vi "Creation IHM Affiche Result.vi"(8 "error in (no error)":errorcluster caption="entrée d'erreur (pas d'erreur)", 10 "Test Result":T3(array[cluster]), 11 "Arbre Liste SN":refnum<vi>) -> (0 "error out":errorcluster caption="sortie d'erreur")   [LabVIEW 2020, in "Library Instrument & Equipement.lvlib" / "Library Popup.lvlib" / "Class Popup Result_Info (Virtual).lvclass"]
uses:
  Class Popup Result_Info (Virtual).lvclass
  Commun VI/TypeDef/Commande Test/Commande Value Type.ctl
  Commun VI/TypeDef/Commande Test/Commande Type Test.ctl
  Commun VI/Library Commun.lvlib
panel:
  in  "Tableau élément":T4(array[cluster])
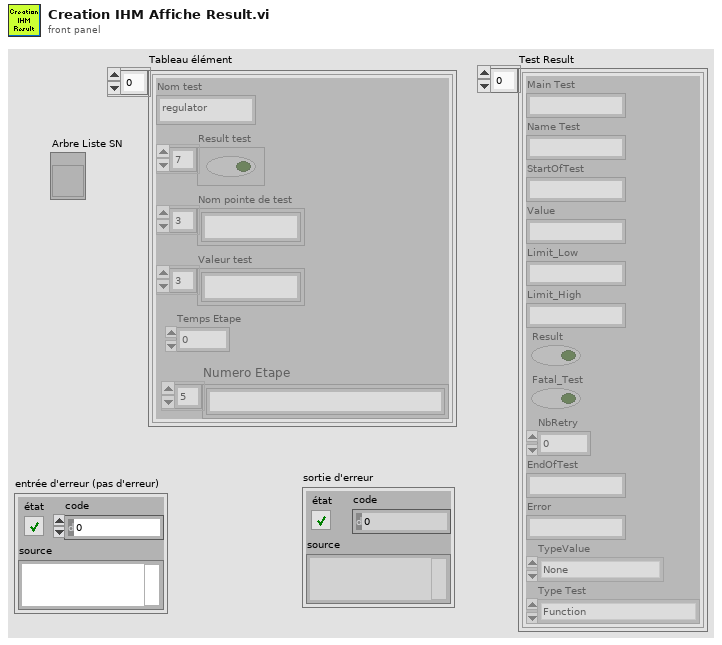
[diagram p1: front panel]
types:
  T1 = typedef "Library Commun.lvlib/Commande Value Type.ctl" = enum16{"None", "String", "Number", "Timestamp", "Boolean", "Array"}
  T2 = typedef "Library Commun.lvlib/Commande Type Test.ctl" = enum16{"Function", "Test", "Calculation"}
  T3 = cluster{"Main Test":string, "Name Test":string, "StartOfTest":string, "Value":string, "Limit_Low":string, "Limit_High":string, "Result":bool, "Fatal_Test":bool, "NbRetry":dbl, "EndOfTest":string, "Error":string, "TypeValue":T1, "Type Test":T2}[]
  T4 = cluster{"Nom test":string, "Result test":bool[], "Nom pointe de test":string[], "Valeur test":string[], "Temps Etape":dbl, "Numero Etape":string[]}[]
  T5 = cluster{"Main Test":string, "Name Test":string, "StartOfTest":string, "Value":string, "Limit_Low":string, "Limit_High":string, "Result":bool, "Fatal_Test":bool, "NbRetry":dbl, "EndOfTest":string, "Error":string, "TypeValue":T1, "Type Test":T2}
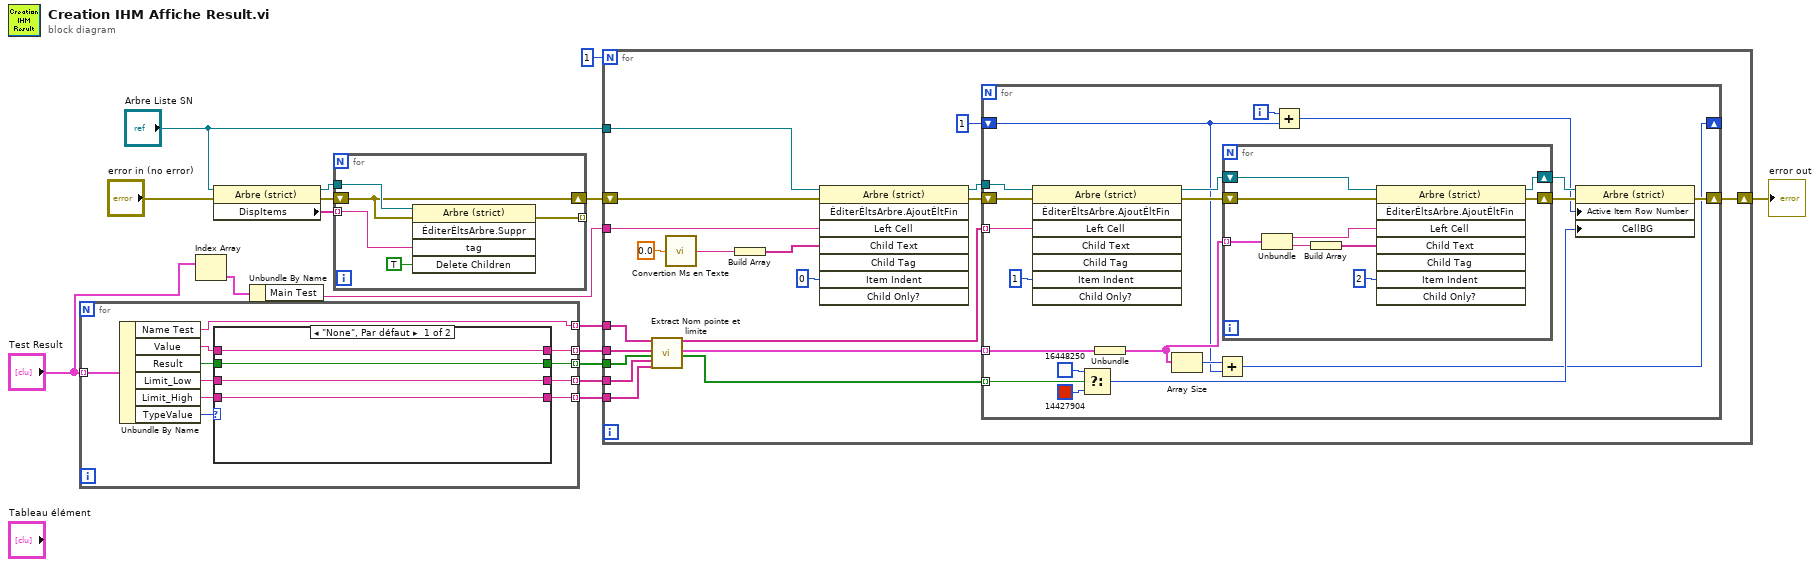
[diagram p0: block diagram]
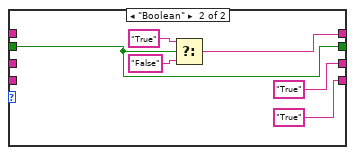
[diagram p2: hidden frame]
diagram:
  n1 = for {
    tunnel: "Test Result" -> [w27] mode=indexing
    tunnel: [w26] -> w9 mode=indexing
    tunnel: [w23] -> w8 mode=indexing
    tunnel: [w17] -> w7 mode=indexing
    tunnel: [w21] -> w6 mode=indexing
    tunnel: [w19] -> w5 mode=indexing
    n2 = Unbundle By Name(w27) -> ("Name Test"=w26:string, "Value"=w24:string, "Result"=w18:bool, "Limit_Low"=w22:string, "Limit_High"=w20:string, "TypeValue"=w25:T1)
    n3 = case shown="\"None\", Par défaut" w25 {
      tunnel: w24 -> [w31 _]
      tunnel: [w31 w35] -> w23
      tunnel: w18 -> [w28 w34]
      tunnel: w22 -> [w30 _]
      tunnel: w20 -> [w29 _]
      tunnel: [w30 "True" ("Limit_Low")] -> w21
      tunnel: [w29 "True" ("Limit_High")] -> w19
      tunnel: [w28 w34] -> w17
      frame "None", Default {
      }
      frame "Boolean" {
        n4 = Select(t="True", s=w34, f="False" ("cas faux")) -> (s? t:f=w35:string)
      }
    }
  }
  n5 = Index Array(array="Test Result") -> (element=w3:T5)  [unwired: 1 in]
  n6 = property class="Arbre (strict)"(reference="Arbre Liste SN", error in="error in (no error)") -> (reference out=w15:refnum<vi>, error out=w14:errorcluster, "DispItems"=w16:string[])
  n7 = Unbundle By Name(w3) -> ("Main Test"=w2:string)
  n8 = for {
    shift-right: [w38] -> w13
    shift-left: w14 -> [w38]
    tunnel: w16 -> [w42] mode=indexing
    tunnel: w15 -> [w41]
    tunnel: [w39] -> _ mode=indexing
    n9 = invoke class="Arbre (strict)" method="ÉditerÉltsArbre.Suppr"(reference=w41, error in=w38, "tag"=w42, "Delete Children"=TRUE ("Supprimer les enfants ?")) -> (error out=w39:errorcluster)  [unwired: 1 in, 4 out]
  }
  n10 = for {
    N: 1 -> [_]
    tunnel: "Arbre Liste SN" -> [w54]
    shift-right: [w57] -> w12
    shift-left: w13 -> [w58]
    tunnel: w9 -> [w49]
    tunnel: w8 -> [w48]
    tunnel: w7 -> [w47]
    tunnel: w6 -> [w45]
    tunnel: w5 -> [w44]
    tunnel: w2 -> [w43]
    n11 = call "Extract Nom pointe et limite.vi"("Nom pointe de test"=w49, "Valeur test"=w48, "Result test"=w47, "Limit Low"=w45, "Limit High"=w44) -> ("Nom test"=w55:string[], "Enfant"=w56:cluster{cluster{"élément":string, string}[]}[], "Result test"=w51:bool[])  [unwired: 12 in]
    n12 = call "Convertion Ms en Texte.vi"("Numérique"=0.0) -> ("Chaîne"=w53:string)
    n13 = Build Array(w53) -> (w52:string[])
    n14 = invoke class="Arbre (strict)" method="ÉditerÉltsArbre.AjoutÉltFin"(reference=w54, error in=w58, "Left Cell"=w43, "Child Text"=w52, "Item Indent"=0 ("Indentation du nouvel élément")) -> (reference out=w59:refnum<vi>, error out=w60:errorcluster)  [unwired: 3 in, 6 out]
    n15 = for {
      tunnel: w55 -> [w79] mode=indexing
      shift-right: [w74] -> w57
      shift-left: w60 -> [w81]
      tunnel: w59 -> [w78]
      tunnel: w51 -> [w77] mode=indexing
      tunnel: w56 -> [w68] mode=indexing
      shift-right: [w62] -> _
      shift-left: 1 ("y") -> [w63]
      i -> [w67]
      n16 = invoke class="Arbre (strict)" method="ÉditerÉltsArbre.AjoutÉltFin"(reference=w78, error in=w81, "Left Cell"=w79, "Item Indent"=1 ("Indentation du nouvel élément")) -> (reference out=w72:refnum<vi>, error out=w70:errorcluster)  [unwired: 4 in, 6 out]
      n17 = Select(t=u32 16448250, s=w77, f=u32 14427904) -> (s? t:f=w73:u32)
      n18 = Unbundle(w68) -> (w65:cluster{"élément":string, string}[])
      n19 = Array Size(array=w65) -> (size(s)=w64:i32)
      n20 = Add(x=w64, y=w63) -> (x+y=w62:i32)
      n21 = for {
        shift-right: [w89] -> w71
        shift-left: w72 -> [w90]
        shift-right: [w87] -> w69
        shift-left: w70 -> [w88]
        tunnel: w65 -> [w85] mode=indexing
        n22 = Unbundle(w85) -> ("élément"=w84:string, w83:string)
        n23 = Build Array(w83) -> (w82:string[])
        n24 = invoke class="Arbre (strict)" method="ÉditerÉltsArbre.AjoutÉltFin"(reference=w90, error in=w88, "Left Cell"=w84, "Child Text"=w82, "Item Indent"=2 ("Indentation du nouvel élément")) -> (reference out=w89:refnum<vi>, error out=w87:errorcluster)  [unwired: 3 in, 6 out]
      }
      n25 = Add(x=w67, y=w63) -> (x+y=w66:i32)
      n26 = property class="Arbre (strict)"(reference=w71, error in=w69, "Active Item Row Number"=w66, "CellBG"=w73) -> (error out=w74:errorcluster)  [unwired: 1 out]
    }
  }
  "error out" <- w12
